vi "Set FileMask.vi"(8 "error in (no error)":errorcluster, 10 "FileMask":string, 11 "TransferFolder in":refnum<class "TransferFolder.lvclass">) -> (0 "error out":errorcluster, 3 "TransferFolder out":refnum<class "TransferFolder.lvclass">)   [LabVIEW 2015, in "WinSCP.lvlib" / "TransferFolder.lvclass"]
uses:
  TransferFolder.lvclass
  TransferFolder.lvclass/TransferFolder.ctl
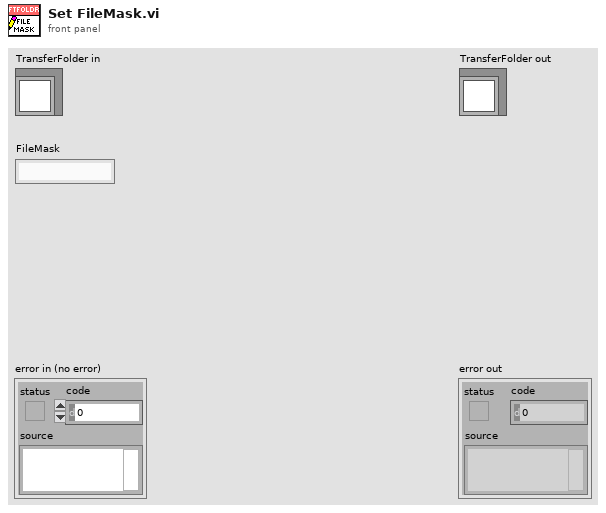
[diagram p1: front panel]
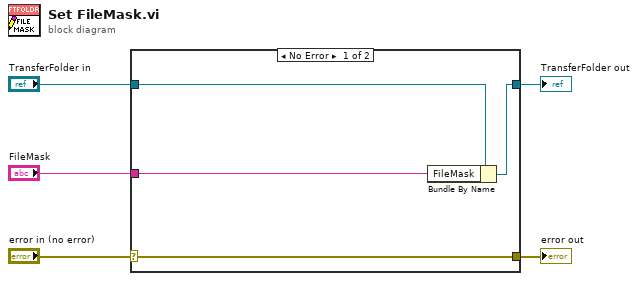
[diagram p0: block diagram]
diagram:
  n1 = case shown="No Error" "error in (no error)" {
    selector: "error in (no error)" -> [w9 w10]
    tunnel: [w9 w10] -> w4
    tunnel: [w7 w11] -> w2
    tunnel: "TransferFolder in" -> [w8 w11]
    tunnel: "FileMask" -> [w6 _]
    frame No Error {
      n2 = Bundle By Name(cluster=w8, "FileMask"=w6) -> (w7:refnum<class "TransferFolder.lvclass">)
    }
    frame Error {
    }
  }
  "error out" <- w4
  "TransferFolder out" <- w2
